vi "ExtraDownsample.vi"(4 "CIC Gain":fxp<+/-,32,1>=0.00390625 format="%#_32g", 6 "Set downsample":bool, 7 "reset":bool, 8 "valid in":bool, 9 "Downsample":fxp<+,8,8>, 10 "I in":fxp<+/-,16,14>, 11 "Q in":fxp<+/-,16,14>) -> (0 "valid out":bool, 2 "Q out":fxp<+/-,16,14>, 3 "I out":fxp<+/-,16,14>)   [LabVIEW 2013]
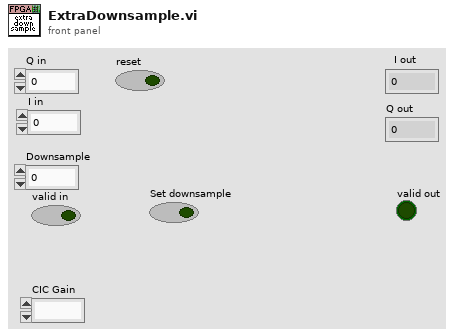
[diagram p1: front panel]
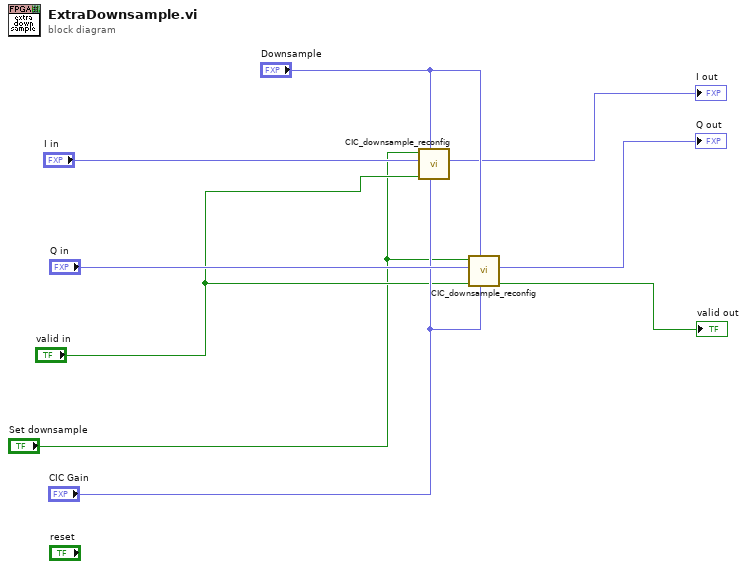
[diagram p0: block diagram]
diagram:
  n1 = call "CIC_downsample_reconfig.vi"("Gain"="CIC Gain", "new rate"="Downsample", "valid in"="valid in", "Data in"="I in", "rate change"="Set downsample") -> ("dout"=→"I out":fxp<+/-,16,14>)  [unwired: 4 in, 2 out]
  n2 = call "CIC_downsample_reconfig.vi"("Gain"="CIC Gain", "new rate"="Downsample", "valid in"="valid in", "Data in"="Q in", "rate change"="Set downsample") -> ("valid out"=→"valid out":bool, "dout"=→"Q out":fxp<+/-,16,14>)  [unwired: 4 in, 1 out]
